vi "setREF_TC.vi"(8 "error in (no error)":errorcluster, 9 "TC (s)":dbl=1e-05 min=0.0001 format="%#_3p", 10 "REF Channel":T1=1 min=1 max=16, 11 "Instrument.Lockin in":refnum<class "Instrument.Lockin.lvclass">) -> (0 "error out":errorcluster, 3 "Instrument.Lockin out":refnum<class "Instrument.Lockin.lvclass">)   [LabVIEW 2019, in "Instrument.Lockin.lvclass"]
doc: "API to configure a REF frequency.\n\nSpecify which channel you want to change and the value you want to set.\n\nIf address=\"\", this API reads from localhost\nIf address is remote lockin, you need to add this computer to allowed whitelist on the lockin computer you are trying to access."
uses:
  Instrument.Lockin.lvclass
  Typedefs/API/Lockin.Commands--Enum.ctl
  97eaa401-7be6-42d3-beed-c4ab4e0956cc.vi
  Lockin.DAQ/Typedefs/REF_Channel-Numeric.ctl
  Lockin.DAQ/Lockin.DAQ.lvclass
  Typedefs/API/Lockin.setREF_TC--cluster.ctl
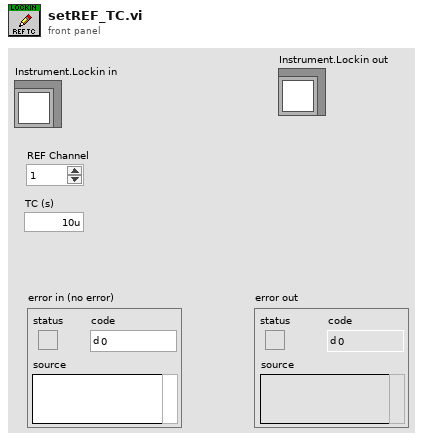
[diagram p1: front panel]
types:
  T1 = typedef "Lockin.DAQ.lvclass/REF_Channel-Numeric.ctl" = i32
  T2 = typedef "Instrument.Lockin.lvclass/Lockin.setREF_TC--cluster.ctl" = cluster{"REF Channel":T1, "TC (s)":dbl}
  T3 = typedef "Instrument.Lockin.lvclass/Lockin.Commands--Enum.ctl" = enum16{"setAO", "setAO_Amplitude", "setAO_DC", "setAO_Frequency", "setAO_Phase", "setAO_Function", "setAO_I+", "setREF", "setREF_Frequency", "setREF_Phase", "setREF_TC", "setREF_Roll-Off", "setIVmode", "setDAQ", "Reset", "setSampling", "setOffset", "Trigger", "getAO", "getAI", "getResults", "getTrigger", "getIVmode", "getSampling", "getAOconfig", "getREFconfig", "setInputGain", "setOutputGain", "getInputGain", "getOutputGain", "setAutoSampling", "getAutoSampling", "setSweep", "getStatus", "getSweepResults", "getSweepWaveforms", "startSweep", "stopSweep", "setAUX", "getAUX", "getRefreshTime"}
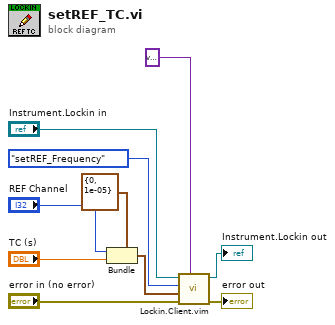
[diagram p0: block diagram]
diagram:
  n1 = Bundle(cluster=T2 {"REF Channel"=0, "TC (s)"=1e-05} ("setREF_phi"), "REF Channel"="REF Channel", "TC (s)"="TC (s)") -> (w4:T2)
  n2 = call "Lockin.Client.vim"("Data Out type"=variant, "error in (no error)"="error in (no error)", "Data"=w4, "Command"=Lockin.Commands--Enum."setREF_Frequency", "Instrument.Lockin in"="Instrument.Lockin in") -> ("error out"=→"error out":errorcluster, "Instrument.Lockin out"=→"Instrument.Lockin out":refnum<class "Instrument.Lockin.lvclass">)  [unwired: 4 in, 1 out]
